vi "Emergency Broadcast.vi"(8 "error in (no error)":errorcluster, 9 "Mail Strategy In":refnum<class "Mail Strategy.lvclass">, 10 "Message In":refnum<class "Message.lvclass">, 11 "Messenger in":refnum<class "Messenger.lvclass">) -> (0 "error out":errorcluster, 3 "Messenger out":refnum<class "Messenger.lvclass">)   [LabVIEW 2024, in "Messenger.lvclass"]
uses:
  Messenger.lvclass
  Message/Message.lvclass
  Mail Strategy/Mail Strategy.lvclass
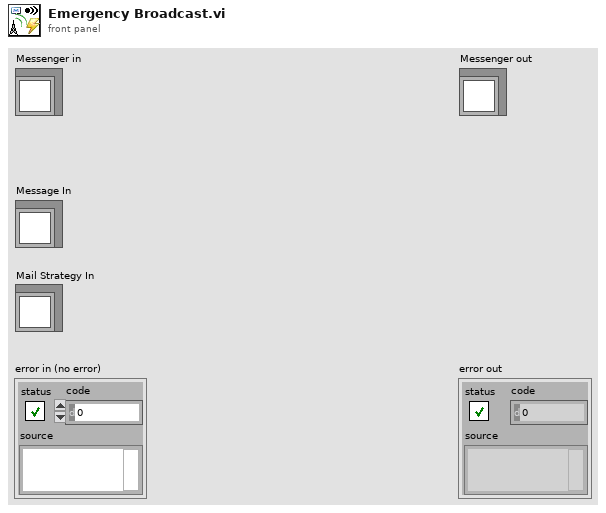
[diagram p1: front panel]
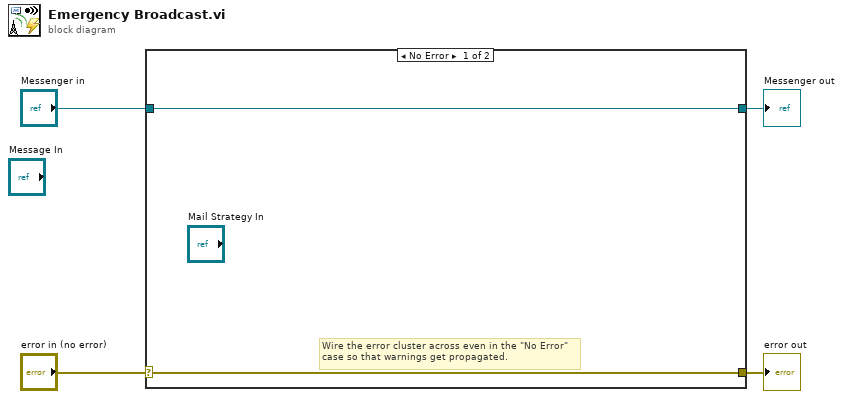
[diagram p0: block diagram]
diagram:
  n1 = case shown="No Error" "error in (no error)" {
    selector: "error in (no error)" -> [w5 w8]
    tunnel: [w5 w8] -> w3
    tunnel: [w6 w7] -> w1
    tunnel: "Messenger in" -> [w6 w7]
    frame No Error {
      # "Wire the error cluster across even in the \"No Error\"\ncase so that warnings get propagated."
    }
    frame Error {
    }
  }
  "error out" <- w3
  "Messenger out" <- w1
